vi "纳清浊度_所有参数读取.vi"(8 "error in (no error)":errorcluster caption="错误输入（无错误）", 11 "MB session in":refnum<class "MB_Master.lvclass">) -> (0 "error out":errorcluster caption="错误输出", 2 "输出值":T1 {"波特率" items=["4800", "9600", "19200", "38400", "57600", "115200"]}, 3 "MB session out":refnum<class "MB_Master.lvclass">)   [LabVIEW 2022 SP3, in "斯坦道多参数.lvlib"]
uses:
  <vilib>/Plasmionique/MB Master/MB_Master/MB_Master.lvclass
  <vilib>/Plasmionique/MB Master/MB Master.lvlib
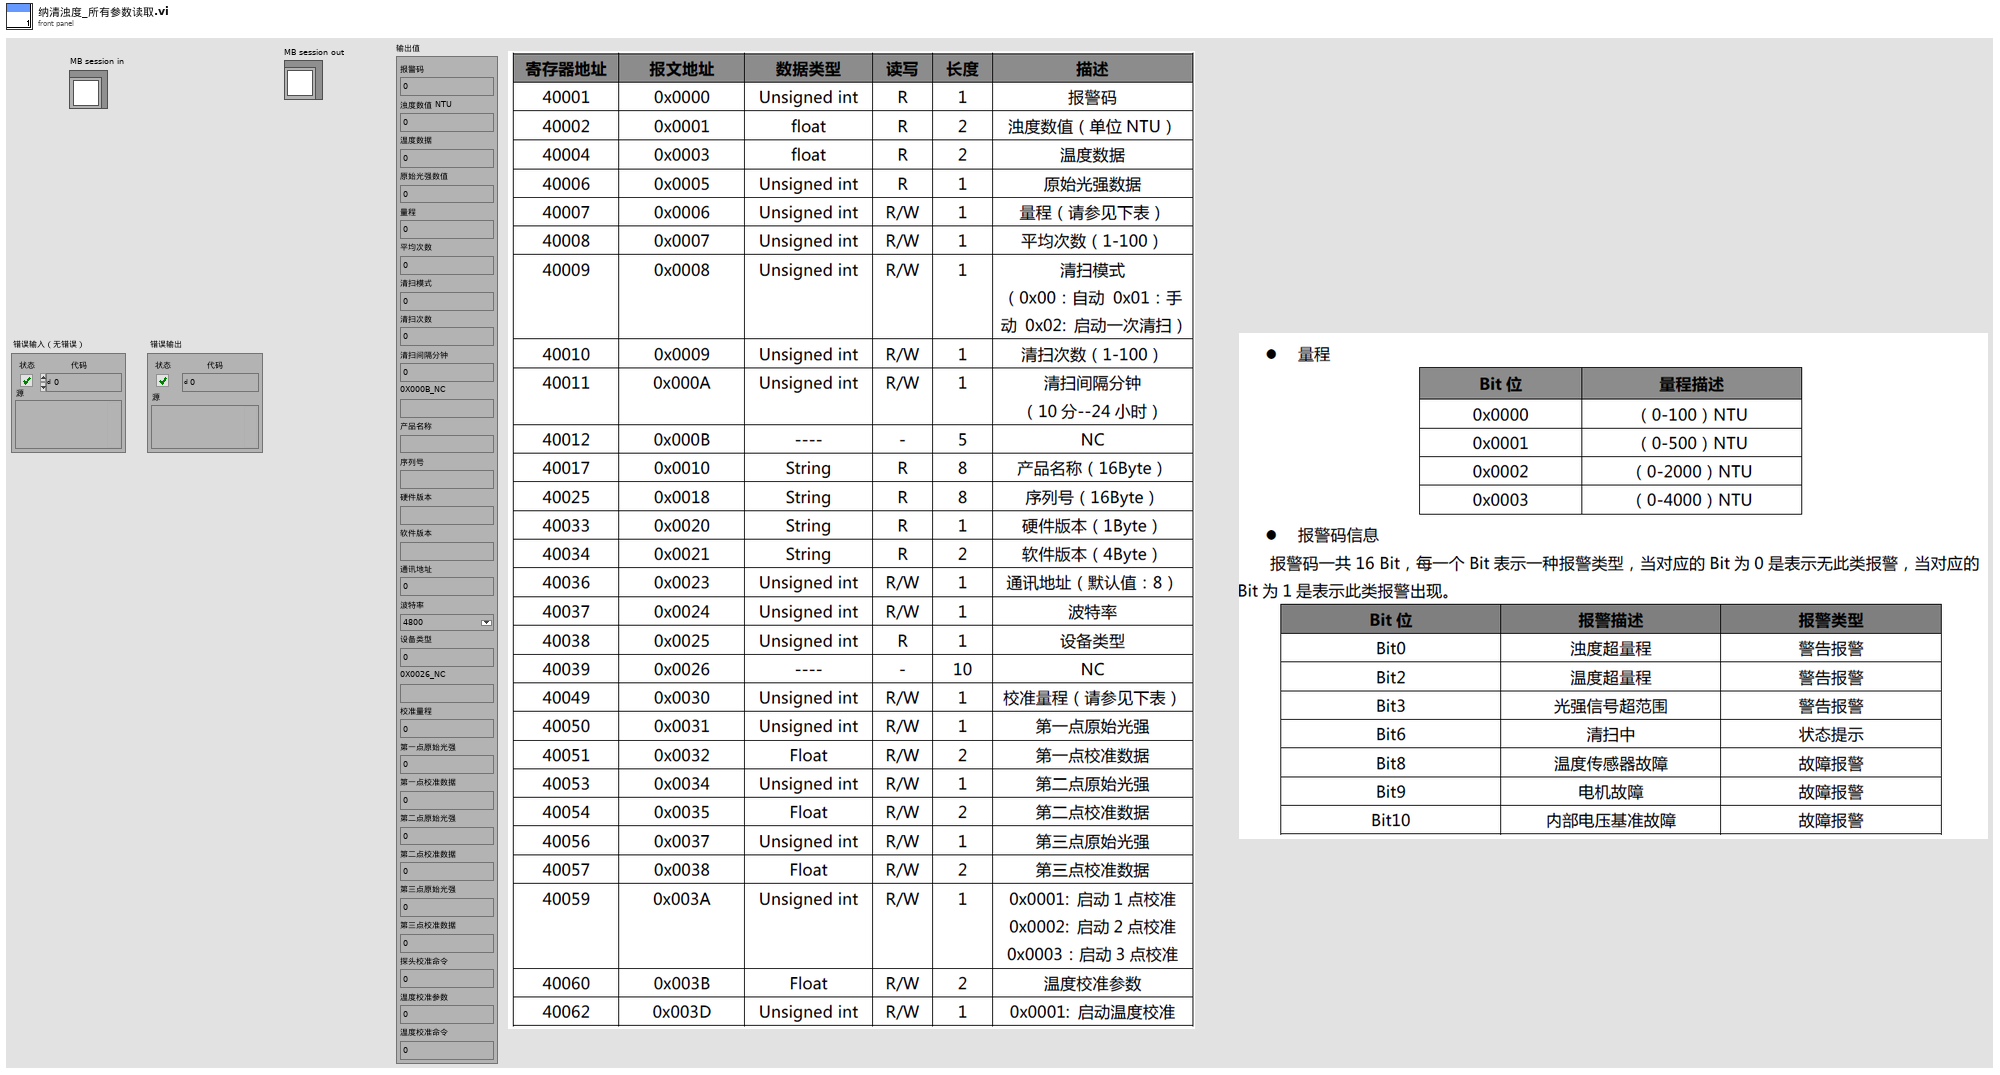
[diagram p1: front panel]
types:
  T1 = cluster{"报警码":u16, "浊度数值 NTU":sgl, "温度数据":sgl, "原始光强数值":u16, "量程":u16, "平均次数":u16, "清扫模式":u16, "清扫次数":u16, "清扫间隔分钟":u16, "0X000B_NC":string, "产品名称":string, "序列号":string, "硬件版本":string, "软件版本":string, "通讯地址":u16, "波特率":u16, "设备类型":u16, "0X0026_NC":string, "校准量程":u16, "第一点原始光强":u16, "第一点校准数据":sgl, "第二点原始光强":u16, "第二点校准数据":sgl, "第三点原始光强":u16, "第三点校准数据":sgl, "探头校准命令":u16, "温度校准参数":sgl, "温度校准命令":u16}
  T2 = cluster{"pH":u32, "DO":u32, "Cond":u32, "Turb":u32, "叶绿素a":u32, "藻密度":u32, "ORP":u32, "COD":u32, "氯化物":u32, "氨氮":u32, "水中油":u32, "悬浮物":u32, "余氯":u32}
  T3 = cluster{u16, "mode":dbl, "数值":sgl, u16, u16, u16, u16, u16, u16, "类型":string, "类型":string, "类型":string, "类型":string, "类型":string, u16, u16, u16, "类型":string, u16, u16, "数值":sgl, u16, "数值":sgl, u16, "数值":sgl, u16, "数值":sgl, u16}
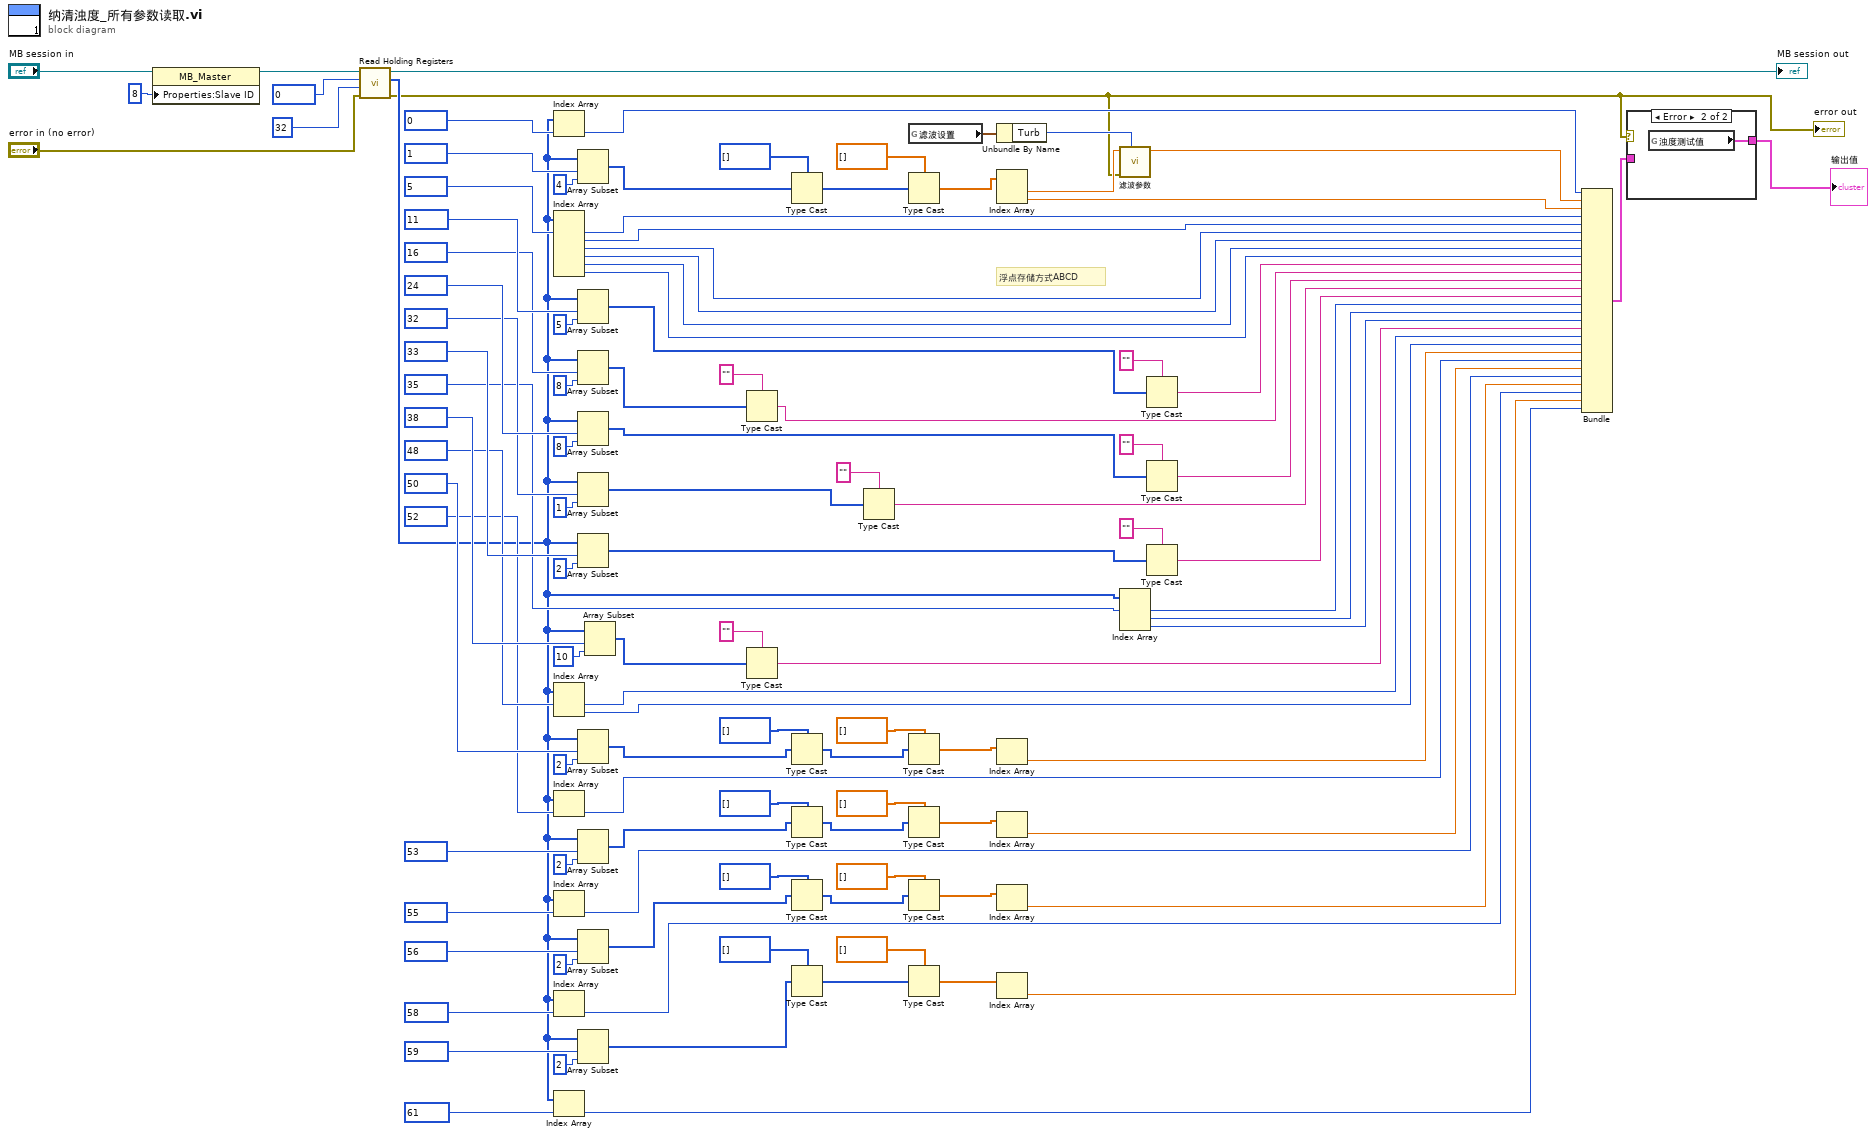
[diagram p0: block diagram]
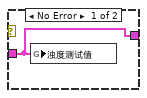
[diagram p2: hidden frame]
diagram:
  # "浮点存储方式ABCD"
  n1 = property class="MB_Master"(reference="MB session in", "Properties:Slave ID"=u8 8 ("Slave ID")) -> (reference out=w99:refnum<class "MB_Master.lvclass">)  [unwired: 1 in, 1 out]
  n2 = call <vilib>:"Read Holding Registers.vi"("error in (no error)"="error in (no error)", "quantity"=u16 32, "starting address"=u16 0, "MB session in"=w99) -> ("error out"=w1:errorcluster, "Registers"=w2:u16[], "MB session out"=→"MB session out":refnum<class "MB_Master.lvclass">)  [unwired: 5 in]
  "error out" <- w1
  n3 = Index Array(array=w2, index=u16 0 ("starting address")) -> (element=w107:u16)
  n4 = Index Array(array=w2, index #1=u16 5 ("starting address")) -> (element #1=w94:u16, element #2=w93:u16, element #3=w92:u16, element #4=w91:u16, element #5=w90:u16, element #6=w89:u16)  [unwired: 5 in]
  n5 = Index Array(array=w2, index #1=u16 48 ("starting address")) -> (element #1=w53:u16, element #2=w52:u16)  [unwired: 1 in]
  n6 = Index Array(array=w2, index=u16 52 ("starting address")) -> (element=w35:u16)
  n7 = Index Array(array=w2, index=u16 55 ("starting address")) -> (element=w25:u16)
  n8 = Index Array(array=w2, index=u16 58 ("starting address")) -> (element=w15:u16)
  n9 = Index Array(array=w2, index=u16 61 ("starting address")) -> (element=w12:u16)
  n10 = Array Subset(array=w2, index=u16 1 ("starting address"), length=4 ("长度")) -> (w103:u16[])
  n11 = Array Subset(array=w2, index=u16 11 ("starting address"), length=5 ("长度")) -> (w86:u16[])
  n12 = Array Subset(array=w2, index=u16 16 ("starting address"), length=8 ("长度")) -> (w82:u16[])
  n13 = Array Subset(array=w2, index=u16 24 ("starting address"), length=8 ("长度")) -> (w76:u16[])
  n14 = Array Subset(array=w2, index=u16 32 ("starting address"), length=1 ("长度")) -> (w72:u16[])
  n15 = Array Subset(array=w2, index=u16 33 ("starting address"), length=2 ("长度")) -> (w66:u16[])
  n16 = Array Subset(array=w2, index=u16 50 ("starting address"), length=2 ("长度")) -> (w50:u16[])
  n17 = Array Subset(array=w2, index=u16 53 ("starting address"), length=2 ("长度")) -> (w38:u16[])
  n18 = Array Subset(array=w2, index=u16 56 ("starting address"), length=2 ("长度")) -> (w31:u16[])
  n19 = Array Subset(array=w2, index=u16 59 ("starting address"), length=2 ("长度")) -> (w18:u16[])
  n20 = Array Subset(array=w2, index=u16 38 ("starting address"), length=10 ("长度")) -> (w56:u16[])
  n21 = Type Cast(type="" ("类型"), x=w82) -> (*(type *) &x=w79:string)
  n22 = Type Cast(type="" ("类型"), x=w56) -> (*(type *) &x=w55:string)
  n23 = Type Cast(type=u32[] [] ("数组 2"), x=w103) -> (*(type *) &x=w10:u32[])
  n24 = Type Cast(type=u32[] [] ("数组 2"), x=w50) -> (*(type *) &x=w48:u32[])
  n25 = Type Cast(type=u32[] [] ("数组 2"), x=w38) -> (*(type *) &x=w40:u32[])
  n26 = Type Cast(type=u32[] [] ("数组 2"), x=w31) -> (*(type *) &x=w29:u32[])
  n27 = Type Cast(type=u32[] [] ("数组 2"), x=w18) -> (*(type *) &x=w20:u32[])
  n28 = Type Cast(type="" ("类型"), x=w72) -> (*(type *) &x=w69:string)
  n29 = global read "断电保存变量.vi" "滤波设置"() -> (w6:T2)
  n30 = Type Cast(type=sgl[] [] ("数组 2"), x=w10) -> (*(type *) &x=w102:sgl[])
  n31 = Type Cast(type=sgl[] [] ("数组 2"), x=w48) -> (*(type *) &x=w45:sgl[])
  n32 = Type Cast(type=sgl[] [] ("数组 2"), x=w40) -> (*(type *) &x=w43:sgl[])
  n33 = Type Cast(type=sgl[] [] ("数组 2"), x=w29) -> (*(type *) &x=w26:sgl[])
  n34 = Type Cast(type=sgl[] [] ("数组 2"), x=w20) -> (*(type *) &x=w23:sgl[])
  n35 = Unbundle By Name(w6) -> ("Turb"=w5:u32)
  n36 = Index Array(array=w102) -> (element #1=w8:sgl, element #2=w97:sgl)  [unwired: 2 in]
  n37 = Index Array(array=w45) -> (element=w44:sgl)  [unwired: 1 in]
  n38 = Index Array(array=w43) -> (element=w34:sgl)  [unwired: 1 in]
  n39 = Index Array(array=w26) -> (element=w24:sgl)  [unwired: 1 in]
  n40 = Index Array(array=w23) -> (element=w14:sgl)  [unwired: 1 in]
  n41 = call "滤波参数.vi"("滤波次数"=w5, "error in (no error)"=w1, "x"=w8) -> ("mode"=w7:dbl)  [unwired: 7 in, 1 out]
  n42 = Index Array(array=w2, index #1=u16 35 ("starting address")) -> (element #1=w62:u16, element #2=w61:u16, element #3=w60:u16)  [unwired: 2 in]
  n43 = Type Cast(type="" ("类型"), x=w86) -> (*(type *) &x=w84:string)
  n44 = Type Cast(type="" ("类型"), x=w76) -> (*(type *) &x=w74:string)
  n45 = Type Cast(type="" ("类型"), x=w66) -> (*(type *) &x=w64:string)
  n46 = Bundle(w107, "mode"=w7, "数值"=w97, w94, w93, w92, w91, w90, w89, "类型"=w84, "类型"=w79, "类型"=w74, "类型"=w69, "类型"=w64, w62, w61, w60, "类型"=w55, w53, w52, "数值"=w44, w35, "数值"=w34, w25, "数值"=w24, w15, "数值"=w14, w12) -> (w11:T3)  [unwired: 1 in]
  n47 = case shown="Error" w1 {
    tunnel: w11 -> [w110 _]
    tunnel: [w110 w111] -> w4
    frame No Error {
      n48 = global write "纳清过程全局变量.vi" "浊度测试值"(w110) -> ()
    }
    frame Error {
      n49 = global read "纳清过程全局变量.vi" "浊度测试值"() -> (w111:T1)
    }
  }
  "输出值" <- w4
